vi "Convert keyboard to teleop command.vi"(8 "error in (no error)":errorcluster, 10 "Teleop command in":T1, 11 "Keyboard in":refnum<k1>) -> (0 "error out":errorcluster, 2 "Teleop command out":T1, 3 "Keyboard out":refnum<k1>)   [LabVIEW 2012]
uses:
  Teleop command.ctl
  <vilib>/Utility/inputDevices.llb/keyboardAcquire.vi
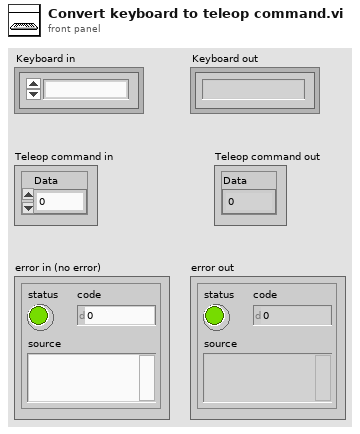
[diagram p1: front panel]
types:
  T1 = typedef "Teleop command.ctl" = cluster{"Data":dbl}
  T2 = enum16{"0", "1", "2", "3", "4", "5", "6", "7", "8", "9", "A", "B", "C", "D", "E", "F", "G", "H", "I", "J", "K", "L", "M", "N", "O", "P", "Q", "R", "S", "T", "U", "V", "W", "X", "Y", "Z", "F1", "F2", "F3", "F4", "F5", "F6", "F7", "F8", "F9", "F10", "F11", "F12", "F13", "F14", "F15", "ADD", "BACK", "BACKSLASH", "CAPITAL", "COMMA", "DECIMAL", "DELETE", "DIVIDE", "DOWN", "END", "EQUALS", "ESCAPE", "GRAVE (`)", "HOME", "INSERT", "LBRACKET", "LCONTROL", "LEFT", "L ALT", "LSHIFT", "LWIN", "MINUS", "MULTIPLY", "NEXT", "NUMLOCK", "NUMPAD_0", "NUMPAD_1", "NUMPAD_2", "NUMPAD_3", "NUMPAD_4", "NUMPAD_5", "NUMPAD_6", "NUMPAD_7", "NUMPAD_8", "NUMPAD_9", "PAUSE", "PERIOD", "PRIOR (PG UP)", "RBRACKET", "RCONTROL", "RETURN", "RIGHT", "R ALT", "RSHIFT", "RWIN", "SCROLL", "SEMICOLON", "SLASH", "SPACE", "SUBTRACT", "TAB", "UP", "ENTER (num pad)", "' (quote)"}[]
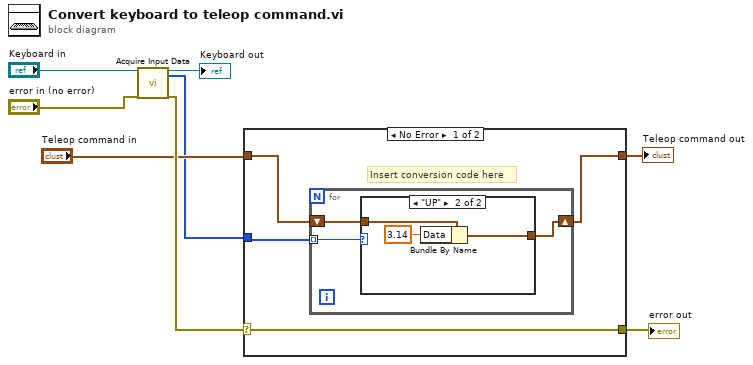
[diagram p0: block diagram]
diagram:
  n1 = call-poly <vilib>:"Acquire Input Data.vi"("device ID"="Keyboard in", "error in (no error)"="error in (no error)") -> ("device ID"=→"Keyboard out":refnum<k1>, "keys pressed"=w1:T2, "error out"=w5:errorcluster)  [unwired: 15 in]
  n2 = case shown="No Error" w5 {
    selector: w5 -> [w12 w21]
    tunnel: [w12 w21] -> w3
    tunnel: "Teleop command in" -> [w10 w20]
    tunnel: [w9 w20] -> w2
    tunnel: w1 -> [w11 _]
    frame No Error {
      # "Insert conversion code here"
      n3 = for {
        tunnel: w11 -> [w15] mode=indexing
        shift-right: [w13] -> w9
        shift-left: w10 -> [w14]
        n4 = case shown="\"UP\"" w15 {
          tunnel: w14 -> [w16 w19]
          tunnel: [w16 w17] -> w13
          frame Default {
          }
          frame "UP" {
            n5 = Bundle By Name(cluster=w19, "Data"=3.14) -> (w17:T1)
          }
        }
      }
    }
    frame Error {
    }
  }
  "Teleop command out" <- w2
  "error out" <- w3
